vi "Update Test Progress.vi"(8 "error in (no error)":errorcluster, 9 "State":string, 10 "Test Name":string, 11 "Test in":refnum<class "Test.lvclass">) -> (0 "error out":errorcluster, 3 "Test out":refnum<class "Test.lvclass">)   [LabVIEW 2017, in "Test.lvlib" / "Test.lvclass"]
uses:
  Test.lvclass
  C:/Program Files (x86)/National Instruments/LabVIEW 2017/vi.lib/ActorFramework/Actor/Actor.lvclass
  <vilib>/ActorFramework/Actor/Actor.lvclass/Actor.ctl
  Test.lvclass/Test.ctl
  Test Messages/Test Progress Msg/Test Progress Msg.lvclass/Test Progress Msg.ctl
  <vilib>/ActorFramework/Message Enqueuer/Message Enqueuer.lvclass/Message Enqueuer.ctl
  <vilib>/ActorFramework/Message Enqueuer/Enqueue.vi
  Test Messages/Test Progress Msg/Test Progress Msg.lvclass
  C:/Program Files (x86)/National Instruments/LabVIEW 2017/vi.lib/ActorFramework/Message/Message.lvclass
  <vilib>/ActorFramework/Message Priority Queue/Priority Enqueue.vi
  <vilib>/ActorFramework/Actor/Actor.lvclass
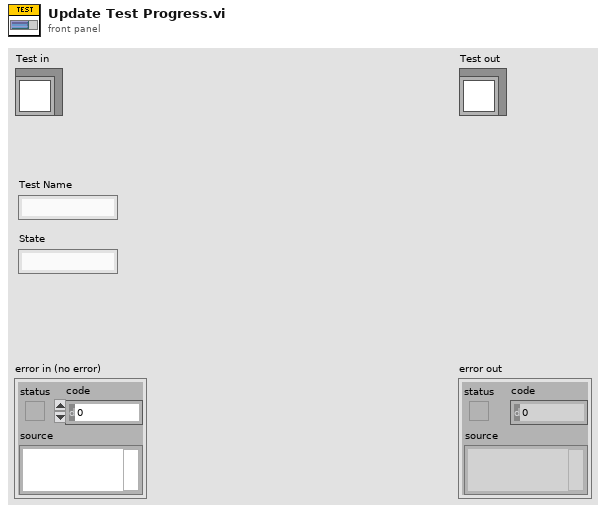
[diagram p1: front panel]
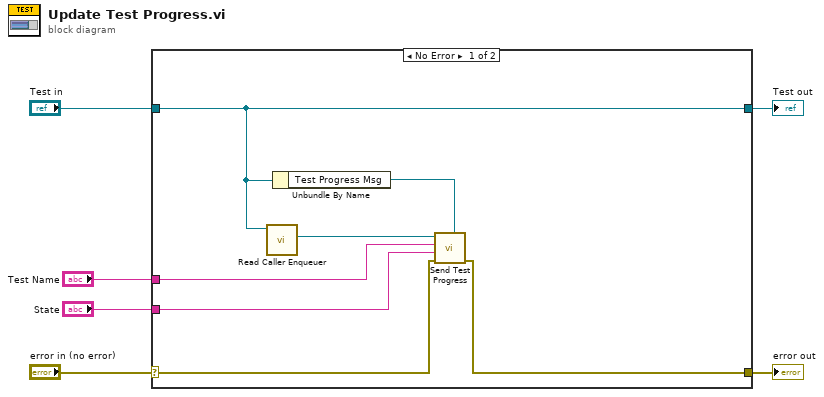
[diagram p0: block diagram]
diagram:
  n1 = case shown="No Error" "error in (no error)" {
    selector: "error in (no error)" -> [w8 w15]
    tunnel: [w7 w15] -> w5
    tunnel: [w12 w14] -> w3
    tunnel: "Test in" -> [w12 w14]
    tunnel: "State" -> [w10 _]
    tunnel: "Test Name" -> [w9 _]
    frame No Error {
      n2 = call <vilib>:"Read Caller Enqueuer.vi"("Actor"=w12) -> ("Caller Enqueuer"=w11:refnum<class "Message Enqueuer.lvclass">)  [unwired: 10 in]
      n3 = Unbundle By Name(w12) -> ("Test Progress Msg"=w13:refnum<class "Test Progress Msg.lvclass">)
      n4 = call "Send Test Progress.vi"("Message Type"=w13, "error in (no error)"=w8, "State"=w10, "Test Name"=w9, "Message Enqueuer"=w11) -> ("error out"=w7:errorcluster)  [unwired: 5 in, 1 out]
    }
    frame Error {
    }
  }
  "error out" <- w5
  "Test out" <- w3
